vi "AI Sample Average (SubVI).vi"(0 "data":dbl[][](array[numeric])) -> (1 "LC_PT_Array":dbl[](array[numeric]), 3 "TC Array":dbl[](array[numeric]))   [LabVIEW 2020]
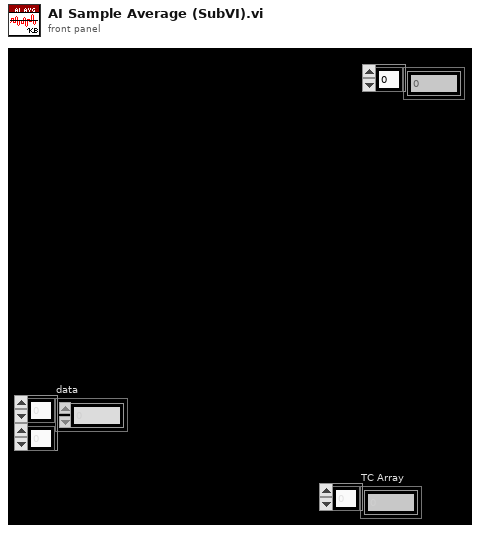
[diagram p1: front panel]
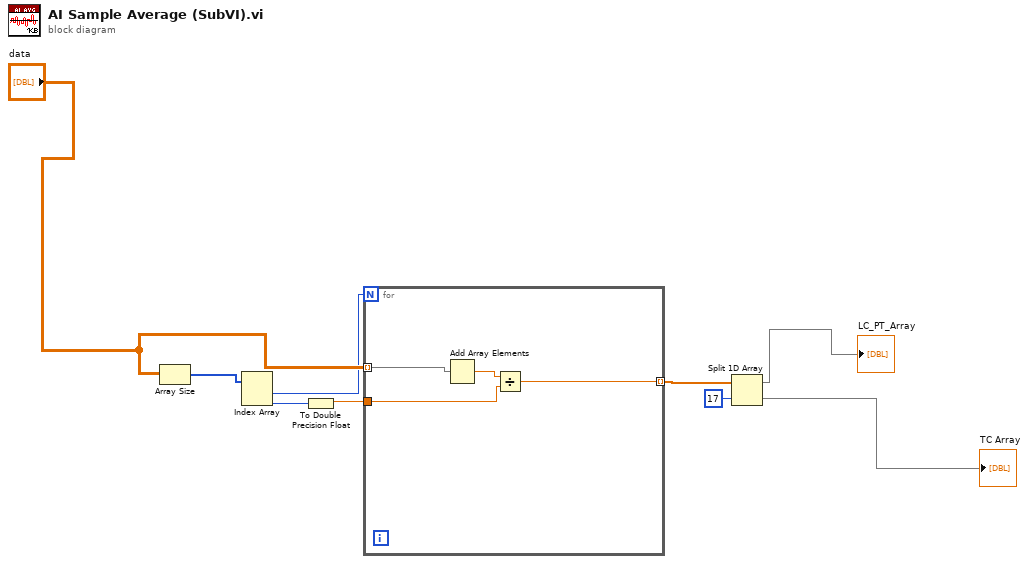
[diagram p0: block diagram]
diagram:
  n1 = Array Size(array="data") -> (size(s)=w8:i32[])
  n2 = Index Array(array=w8) -> (element #1=w5:i32, element #2=w6:i32)  [unwired: 2 in]
  n3 = To Double Precision Float(number=w6) -> (double precision float=w7:dbl)
  n4 = for {
    N: w5 -> [_]
    tunnel: "data" -> [w13] mode=indexing
    tunnel: w7 -> [w11]
    tunnel: [w10] -> w4 mode=indexing
    n5 = Add Array Elements(numeric array=w13) -> (sum=w12:dbl)
    n6 = Divide(x=w12, y=w11) -> (x/y=w10:dbl)
  }
  n7 = Split 1D Array(array=w4, index=17) -> (first subarray=→"LC_PT_Array":dbl[], second subarray=→"TC Array":dbl[])
